vi "Router - Reader.vi"(8 "error in (no error)":errorcluster, 9 "Reading Segments":T1, 10 "PXImc Reading Session In":refnum<k21>, 11 "Master Table Ref In":refnum<data-value>) -> (0 "error out":errorcluster)   [LabVIEW 2016, in "PXImc Router.lvlib"]
uses:
  PXImc Router.lvlib
  Controls/Table Index-Size.ctl
  Router - Globals.vi
  <vilib>/pximc/Acquire Read Region (DBL).vi
  <resource>/objmgr/pximc.rc
  <vilib>/pximc/nipximc.lvlib
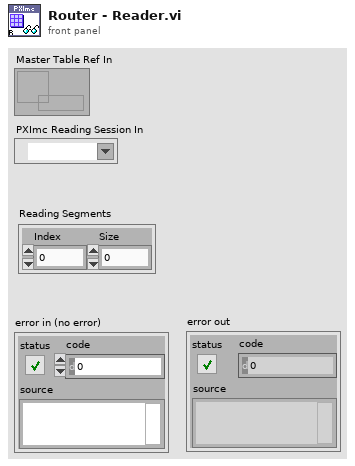
[diagram p1: front panel]
types:
  T1 = typedef "PXImc Router.lvlib/Table Index-Size.ctl" = cluster{"Index":u32, "Size":u32}
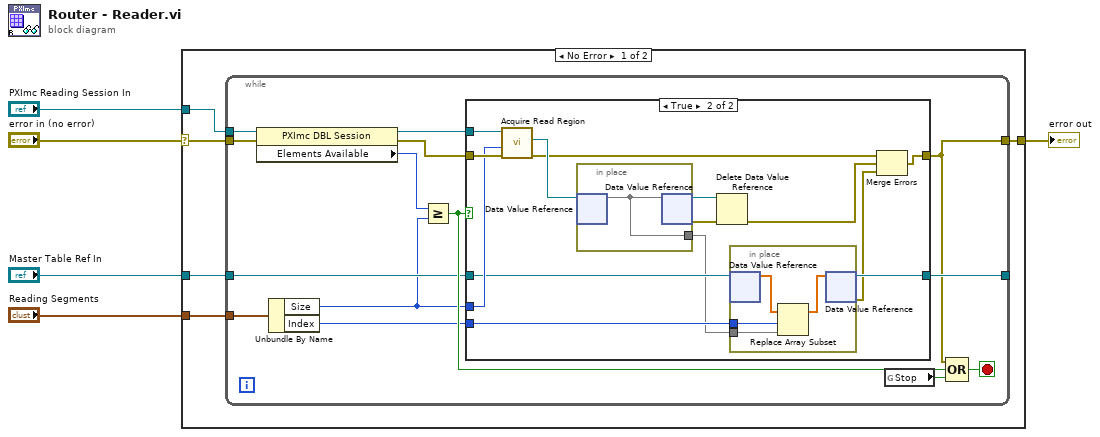
[diagram p0: block diagram]
diagram:
  n1 = case shown="No Error" "error in (no error)" {
    selector: "error in (no error)" -> [w8 w46]
    tunnel: "PXImc Reading Session In" -> [w10 _]
    tunnel: "Master Table Ref In" -> [w9 _]
    tunnel: [w7 w46] -> w4
    tunnel: "Reading Segments" -> [w6 _]
    frame No Error {
      n2 = while {
        tunnel: w10 -> [w24]
        tunnel: w8 -> [w21]
        tunnel: [w14] -> w7
        tunnel: [w19] -> _
        tunnel: w9 -> [w16]
        tunnel: w6 -> [w13]
        stop <- w17 stop-if-true
        n3 = property class="PXImc DBL Session"(reference=w24, error in=w21) -> (reference out=w22:refnum<k21>, error out=w20:errorcluster, "Elements Available"=w23:u64)
        n4 = Unbundle By Name(w13) -> ("Size"=w12:u32, "Index"=w11:u32)
        n5 = Greater Or Equal?(x=w23, y=w12) -> (x >= y?=w18:bool)
        n6 = case shown="True" w18 {
          tunnel: w20 -> [w26 w39]
          tunnel: [w26 w33] -> w14
          tunnel: w22 -> [_ w38]
          tunnel: w11 -> [_ w32]
          tunnel: [w25 w29] -> w19
          tunnel: w12 -> [_ w31]
          tunnel: w16 -> [w25 w30]
          frame False {
          }
          frame True {
            n7 = call-poly <vilib>:"Acquire Read Region.vi"("error in (no error)"=w39, "number of elements"=w31, "session in"=w38) -> ("error out"=w34:errorcluster, "read region reference"=w40:refnum<data-value>)  [unwired: 5 in, 2 out]
            n8 = in-place {
              in-place-border: [w45] -> w28
              n9 = in-place-dvr #1(w40) -> (w45:dbl[])  [unwired: 1 out]
              n10 = in-place-dvr #1(w45) -> (w37:refnum<data-value>, w36:errorcluster)
            }
            n11 = Delete Data Value Reference(data value reference=w37, error in=w36) -> (error out=w35:errorcluster)  [unwired: 1 out]
            n12 = in-place {
              in-place-border: w32 -> [w44]
              in-place-border: w28 -> [w41]
              n13 = in-place-dvr #2(w30) -> (w43:dbl[])  [unwired: 1 out]
              n14 = Replace Array Subset(array=w43, new element=w41, index=w44) -> (w42:dbl[])
              n15 = in-place-dvr #2(w42) -> (w29:refnum<data-value>, w27:errorcluster)
            }
            n16 = Merge Errors(w34, w35, w27) -> (w33:errorcluster)
          }
        }
        n17 = global read "Router - Globals.vi" "Stop"() -> (w15:bool)
        n18 = Compound Arithmetic op=OR(w14, w18, w15) -> (w17:bool)
      }
    }
    frame Error {
    }
  }
  "error out" <- w4
